vi "General Cosine Window (CDB).vi"(2 "Cosine Coefficients":dbl[](array[numeric]), 3 "X":cdb[](array[numeric])) -> (0 "error":i32, 1 "Windowed X":cdb[](array[numeric]))   [LabVIEW 2017, in "NI_AALPro.lvlib"]
doc: "Applies a general cosine window to the input signal <B>X</B>. Wire data to the <B>X</B> input to determine the polymorphic instance to use or manually select the instance."
uses:
  <vilib>/Analysis/NI_AALPro.lvlib
  <resource>/lvanlys.dll
panel:
  # "General Cosine Window"
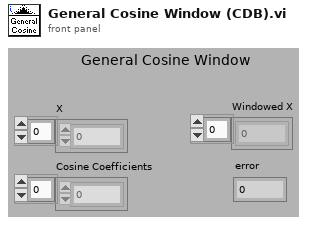
[diagram p1: front panel]
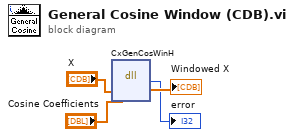
[diagram p0: block diagram]
diagram:
  n1 = dll-call lib="e:/builds/penguin/labview/branches/2017/dev/dist/resource/lvanlys.*" fn="CxGenCosWinH"("X"="X", "Cosine Coefficients"="Cosine Coefficients") -> (→"error":i32, "X"=→"Windowed X":cdb[])  [unwired: 4 in, 2 out]
